vi "MHTML HTML Section.vi"(4 "boundary":string, 7 "file path string":string, 8 "HTML":string) -> (3 "MHTML":string)   [LabVIEW 2011]
panel:
  out "Concatenated String":string
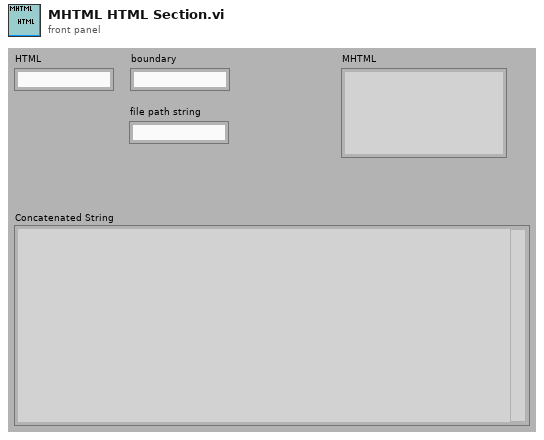
[diagram p1: front panel]
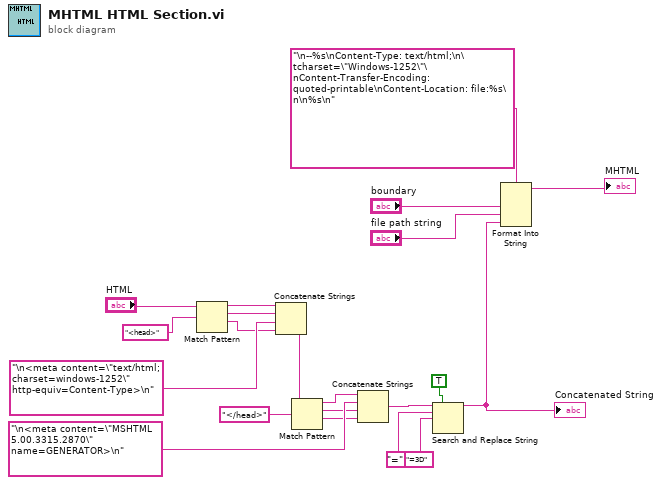
[diagram p0: block diagram]
diagram:
  n1 = Match Pattern(string="HTML", regular expression="<head>") -> (before substring=w15:string, match substring=w14:string, after substring=w12:string)  [unwired: 2 out]
  n2 = Concatenate Strings(w15, w14, "\n<meta content=\"text/html; charset=windows-1252\" http-equiv=Content-Type>\n", w12) -> (w10:string)
  n3 = Match Pattern(string=w10, regular expression="</head>") -> (before substring=w9:string, match substring=w7:string, after substring=w6:string)  [unwired: 2 out]
  n4 = Concatenate Strings(w9, "\n<meta content=\"MSHTML 5.00.3315.2870\" name=GENERATOR>\n", w7, w6) -> (w5:string)
  n5 = Search and Replace String(replace all?=TRUE, input string=w5, search string="=", replace string="=3D") -> (result string=w1:string)  [unwired: 1 in, 6 out]
  "Concatenated String" <- w1
  n6 = Format Into String(format string="\n--%s\nContent-Type: text/html;\n\tcharset=\"Windows-1252\"\nContent-Transfer-Encoding: quoted-printable\nContent-Location: file:%s\n\n%s\n", "boundary", "file path string", w1) -> (resulting string=→"MHTML":string)  [unwired: 2 in, 1 out]
